vi "Test Get Manufacturer Specific Objects.vi"(11 "Test Case In":refnum<class "Test Object Dictionary.lvclass">) -> (0 "error out":errorcluster, 3 "Test Case Out":refnum<class "Test Object Dictionary.lvclass">)   [LabVIEW 2020, in "Test Object Dictionary.lvclass"]
uses:
  Test Object Dictionary.lvclass
  C:/Program Files/National Instruments/LabVIEW 2026/vi.lib/Astemes/LUnit/Test Case.lvclass
  EDS-File-Viewer/source/Electronic Datasheet/Electronic Datasheet.lvclass/Electronic Datasheet.ctl
  source/Object Entry/Object Entry.lvclass/Object Entry.ctl
  source/Sub Object/Sub Object.lvclass/Sub Object.ctl
  <vilib>/Astemes/LUnit/Test Case.lvclass/Test Case.ctl
  source/Sub Object/Sub Object.lvclass
  EDS-File-Viewer/source/Electronic Datasheet/Electronic Datasheet.lvclass
  source/Object Dictionary/Object Dictionary.lvclass
  source/Typedefs/Object Type.ctl
  source/CANopen.lvlib
  <vilib>/Astemes/LUnit/Test Case.lvclass
  source/Object Entry/Object Entry.lvclass
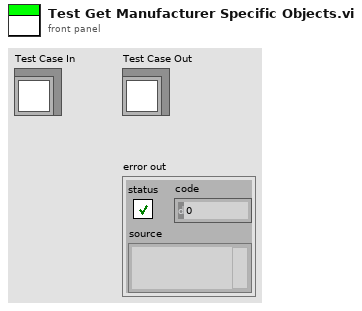
[diagram p1: front panel]
types:
  T1 = typedef "CANopen.lvlib/Object Type.ctl" = u8
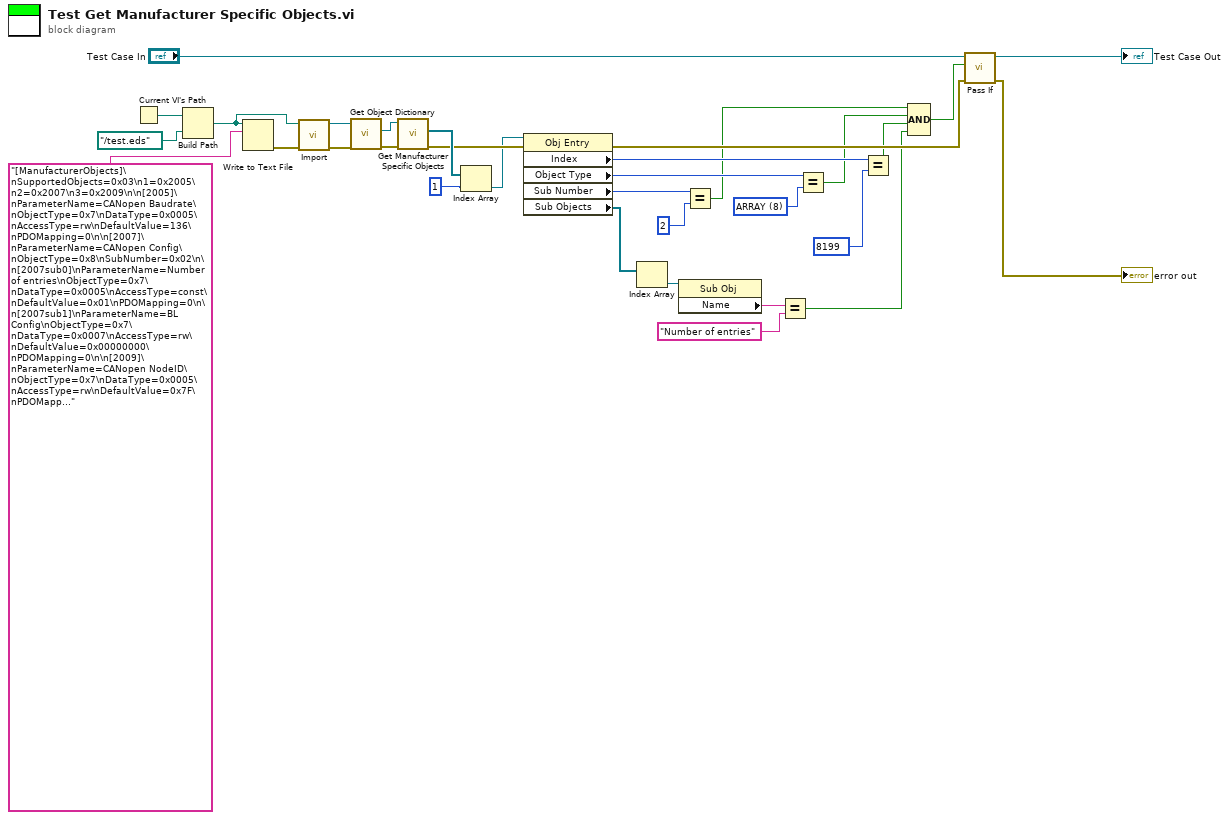
[diagram p0: block diagram]
diagram:
  w15 = T1 8 items=["NULL"=0, "DOMAIN"=2, "DEFTYPE"=5, "DEFSTRUCT"=6, "VAR"=7, "ARRAY"=8, "RECORD"=9] ("y")
  n1 = Current VI's Path() -> (path=w29:path)
  n2 = Build Path(base path=w29, name or relative path=path "../test.eds") -> (appended path=w27:path)
  n3 = Write to Text File(file (use dialog)=w27, text="[ManufacturerObjects]\nSupportedObjects=0x03\n1=0x2005\n2=0x2007\n3=0x2009\n\n[2005]\nParameterName=CANopen Baudrate\nObjectType=0x7\nDataType=0x0005\nAccessType=rw\nDefaultValue=136\nPDOMapping=0\n\n[2007]\nParameterName=CANopen Config\nObjectType=0x8\nSubNumber=0x02\n\n[2007sub0]\nParameterName=Number of entries\nObjectType=0x7\nDataType=0x0005\nAccessType=const\nDefaultValue=0x01\nPDOMapping=0\n\n[2007sub1]\nParameterName=BL Config\nObjectType=0x7\nDataType=0x0007\nAccessType=rw\nDefaultValue=0x00000000\nPDOMapping=0\n\n[2009]\nParameterName=CANopen NodeID\nObjectType=0x7\nDataType=0x0005\nAccessType=rw\nDefaultValue=0x7F\nPDOMapping=0\n") -> (error out=w26:errorcluster)  [unwired: 2 in, 2 out]
  n4 = call "Import.vi"("error in"=w26, "EDS File Path"=w27) -> ("error out"=w25:errorcluster, "Electronic Datasheet"=w24:refnum<class "Electronic Datasheet.lvclass">)  [unwired: 8 in]
  n5 = call "Get Object Dictionary.vi"("error in"=w25, "Electronic Datasheet in"=w24) -> ("error out"=w23:errorcluster, "Obj Dict"=w22:refnum<class "Object Dictionary.lvclass">)  [unwired: 7 in, 1 out]
  n6 = call "Get Manufacturer Specific Objects.vi"("error in"=w23, "Obj Dict in"=w22) -> ("error out"=w19:errorcluster, "Manufacturer Specific"=w21:refnum<class "Object Entry.lvclass">[])  [unwired: 7 in, 1 out]
  n7 = Index Array(array=w21, index=1) -> (element=w17:refnum<class "Object Entry.lvclass">)
  n8 = property class="Obj Entry"(reference=w17, error in=w19) -> (error out=w18:errorcluster, "Index"=w14:u16, "Object Type"=w16:T1, "Sub Number"=w12:u8, "Sub Objects"=w6:refnum<class "Sub Object.lvclass">[])  [unwired: 1 out]
  n9 = Index Array(array=w6) -> (element=w5:refnum<class "Sub Object.lvclass">)  [unwired: 1 in]
  n10 = property class="Sub Obj"(reference=w5) -> ("Name"=w4:string)  [unwired: 1 in, 2 out]
  n11 = Equal?(x=w12, y=u8 2) -> (x = y?=w10:bool)
  n12 = Equal?(x=w4, y="Number of entries") -> (x = y?=w2:bool)
  n13 = Equal?(x=w16, y=w15) -> (x = y?=w9:bool)
  n14 = Equal?(x=w14, y=u16 8199) -> (x = y?=w8:bool)
  n15 = Compound Arithmetic op=AND(w10, w9, w8, w2) -> (w7:bool)
  n16 = call <vilib>:"Pass If.vi"("error in (no error)"=w18, "Pass?"=w7, "LUnit Test Case In"="Test Case In") -> ("error out"=→"error out":errorcluster, "LUnit Test Case Out"=→"Test Case Out":refnum<class "Test Object Dictionary.lvclass">)  [unwired: 7 in]
